vi "workbook set size.vi"(8 "error in (no error)":errorcluster, 9 "height":u16, 10 "width":u16, 11 "workbook":u32) -> (0 "error out":errorcluster)   [LabVIEW 8.6]
doc: "void workbook_set_size(lxw_workbook workbook, uint16_t width, uint16_t height);"
uses:
  pending_lvxlsxwriter/xlsxwriter.dll
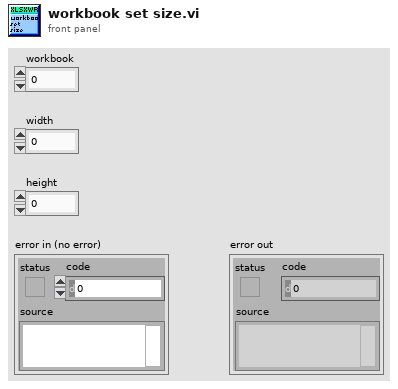
[diagram p1: front panel]
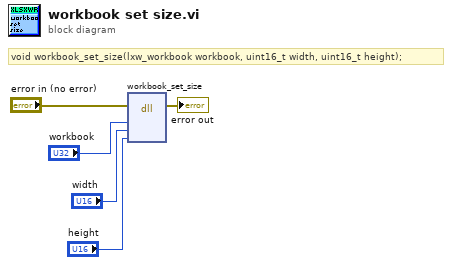
[diagram p0: block diagram]
diagram:
  # "void workbook_set_size(lxw_workbook workbook, uint16_t width, uint16_t height);"
  n1 = dll-call lib="C:/Users/WDAGUtilityAccount/Desktop/pending_lvxlsxwriter/xlsxwriter.*" fn="workbook_set_size"(error in="error in (no error)", "workbook"="workbook", "width"="width", "height"="height") -> (error out=→"error out":errorcluster)  [unwired: 6 in, 1 out]
